vi "sub_GSlam_cal-edges.vi"(10 "z_list":dbl[][][](array[numeric]), 11 "x_list":cluster{"x":dbl, "y":dbl, "yaw":dbl}[](array[cluster])) -> ()   [LabVIEW 2019]
panel:
  in  "cost":dbl
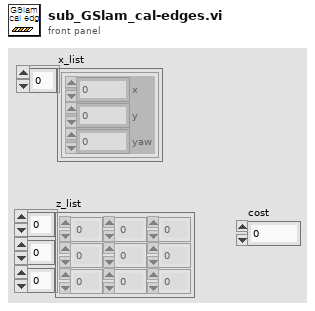
[diagram p1: front panel]
types:
  T1 = cluster{"x_dr":cluster{"x":dbl, "y":dbl, "yaw":dbl}, "x_dr":cluster{"x":dbl, "y":dbl, "yaw":dbl}, "Real Matrix Element":dbl, "Real Matrix Element":dbl, "Real Matrix Element":dbl, "Real Matrix Element":dbl, "x":i32, "y":i32}
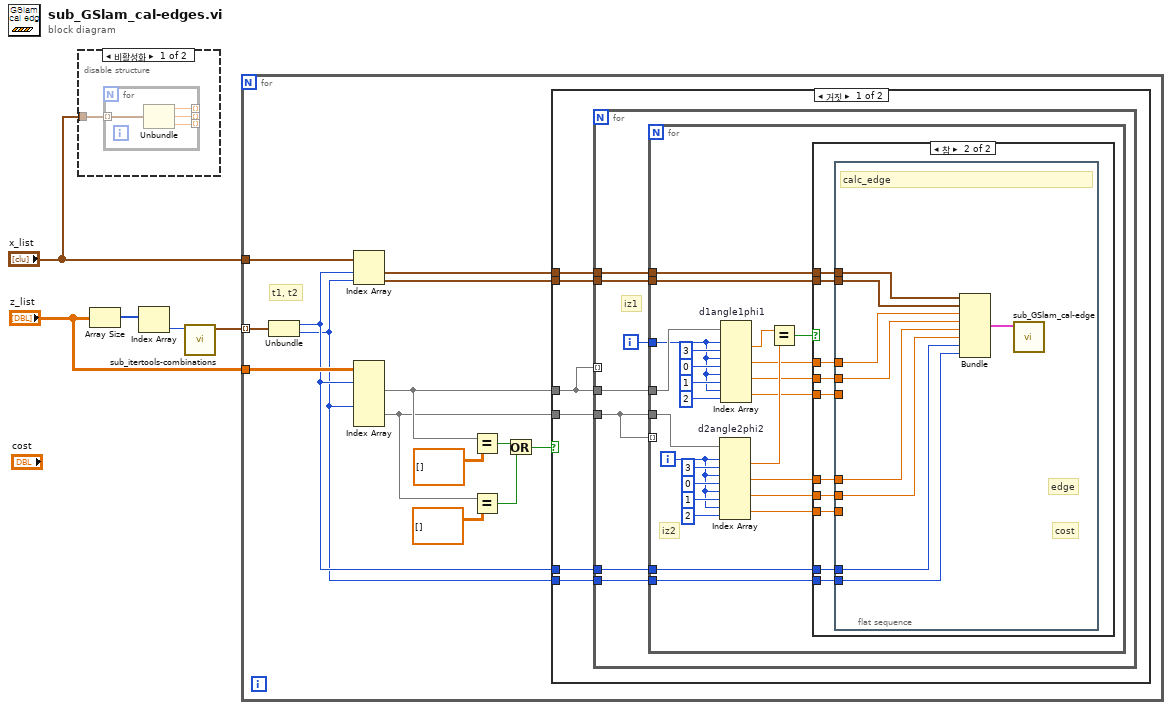
[diagram p0: block diagram]
diagram:
  n1 = disable-structure shown="비활성화" {
    disable-tunnel: "x_list" -> [w6 _]
    frame Disabled {
      n2 = for {
        tunnel: w6 -> [w10] mode=indexing
        tunnel: [w9] -> _ mode=indexing
        tunnel: [w8] -> _ mode=indexing
        tunnel: [w7] -> _ mode=indexing
        n3 = Unbundle(w10) -> ("x"=w9:dbl, "y"=w8:dbl, "yaw"=w7:dbl)
      }
    }
    frame Enabled {
    }
  }
  n4 = Array Size(array="z_list") -> (size(s)=w5:i32[])
  n5 = Index Array(array=w5) -> (element=w4:i32)  [unwired: 1 in]
  n6 = call "sub_itertools-combinations.vi"("N"=w4) -> ("z_ids"=w3:cluster{"x":i32, "y":i32}[])  [unwired: 10 in]
  n7 = for {
    tunnel: w3 -> [w24] mode=indexing
    tunnel: "x_list" -> [w23]
    tunnel: "z_list" -> [w17]
    # "t1, t2"
    n8 = Unbundle(w24) -> ("x"=w12:i32, "y"=w11:i32)
    n9 = Index Array(array=w23, index #1=w12, index #2=w11) -> (element #1=w14:cluster{"x":dbl, "y":dbl, "yaw":dbl}, element #2=w13:cluster{"x":dbl, "y":dbl, "yaw":dbl})
    n10 = Index Array(array=w17, index (dim 0) #1=w12, index (dim 0) #2=w11) -> (element #1=w16:dbl[][], element #2=w15:dbl[][])  [unwired: 4 in]
    n11 = Equal?(x=w16, y=dbl[][] []) -> (x = y?=w18:bool)
    n12 = Equal?(x=w15, y=dbl[][] []) -> (x = y?=w19:bool)
    n13 = Or(x=w18, y=w19) -> (x .or. y?=w20:bool)
    n14 = case shown="거짓" w20 {
      tunnel: w16 -> [w29 _]
      tunnel: w15 -> [w30 _]
      tunnel: w14 -> [w28 _]
      tunnel: w13 -> [w27 _]
      tunnel: w12 -> [w26 _]
      tunnel: w11 -> [w25 _]
      frame False {
        n15 = for {
          tunnel: w29 -> [w37]
          tunnel: w30 -> [w35]
          tunnel: w29 -> [_] mode=indexing
          tunnel: w28 -> [w34]
          tunnel: w27 -> [w33]
          tunnel: w26 -> [w32]
          tunnel: w25 -> [w31]
          i -> [w36]
          # "iz1"
          n16 = for {
            tunnel: w37 -> [w62]
            tunnel: w35 -> [w60]
            tunnel: w36 -> [w47]
            tunnel: w35 -> [_] mode=indexing
            tunnel: w34 -> [w41]
            tunnel: w33 -> [w40]
            tunnel: w32 -> [w39]
            tunnel: w31 -> [w38]
            i -> [w44]
            # "iz2"
            n17 = Index Array "d2angle2phi2"(array=w60, index (row) #1=w44, index (col) #1=3 ("disabled index (col)"), index (row) #2=w44, index (col) #2=0 ("disabled index (col)"), index (row) #3=w44, index (col) #3=1 ("disabled index (col)"), index (row) #4=w44, index (col) #4=2 ("disabled index (col)")) -> (element #1=w58:dbl, element #2=w52:dbl, element #3=w48:dbl, element #4=w42:dbl)
            n18 = Index Array "d1angle1phi1"(array=w62, index (row) #1=w47, index (col) #1=3 ("disabled index (col)"), index (row) #2=w47, index (col) #2=0 ("disabled index (col)"), index (row) #3=w47, index (col) #3=1 ("disabled index (col)"), index (row) #4=w47, index (col) #4=2 ("disabled index (col)")) -> (element #1=w57:dbl, element #2=w54:dbl, element #3=w50:dbl, element #4=w45:dbl)
            n19 = Equal?(x=w57, y=w58) -> (x = y?=w56:bool)
            n20 = case shown="참" w56 {
              tunnel: w54 -> [_ w72]
              tunnel: w52 -> [_ w69]
              tunnel: w50 -> [_ w71]
              tunnel: w48 -> [_ w68]
              tunnel: w45 -> [_ w70]
              tunnel: w42 -> [_ w67]
              tunnel: w41 -> [_ w66]
              tunnel: w40 -> [_ w65]
              tunnel: w39 -> [_ w64]
              tunnel: w38 -> [_ w63]
              frame False {
              }
              frame True {
                n21 = flat-sequence {
                  tunnel: w72 -> [w79]
                  tunnel: w71 -> [w78]
                  tunnel: w70 -> [_]
                  tunnel: w69 -> [w76]
                  tunnel: w68 -> [w77]
                  tunnel: w67 -> [_]
                  tunnel: w66 -> [w81]
                  tunnel: w65 -> [w80]
                  tunnel: w64 -> [w75]
                  tunnel: w63 -> [w74]
                  frame #0 {
                    # "cost"
                    # "edge"
                    # "calc_edge"
                    n22 = Bundle("x_dr"=w81, "x_dr"=w80, "Real Matrix Element"=w79, "Real Matrix Element"=w78, "Real Matrix Element"=w76, "Real Matrix Element"=w77, "x"=w75, "y"=w74) -> (w73:T1)  [unwired: 1 in]
                    n23 = call "sub_GSlam_cal-edge.vi"("in"=w73) -> ()  [unwired: 11 in]
                  }
                }
              }
            }
          }
        }
      }
      frame True {
      }
    }
  }
